vi "ERIO WIN Initialize all Process Variables.vi"(8 "error in (no error)":errorcluster, 9 "Tag Update Values":T1[](array[typedef]), 11 "EEISysLink.lvclass In":refnum<class "EEISysLink.lvclass">) -> (0 "error out":errorcluster, 3 "EEISysLink.lvclass Out":refnum<class "EEISysLink.lvclass">)   [LabVIEW 2017]
doc: "Will initialize all process variables on SystemLink in this ERIO evaluation cloud demo. This includes supervisory and worker types. This prepares the whole demo to run properly. \n\nNOTE: This Windows supervisor program must be run first before the sbRIO process target to properly initialize process variables and enable correct simulation operation. \n\nJames Tillett P.E.\nEndeavor Engineering Inc.\nwww.endeavoreng.com"
uses:
  Class EEISysLink/EEISysLink.lvclass
  Class EEISysLink/Controls/SL Tag Value.ctl
  Class EEISysLink/Controls/SL Tag Data Type.ctl
  Class EEISysLink/Controls/SL Tag Scope.ctl
  Class EEISysLink/Controls/SL Tag Type.ctl
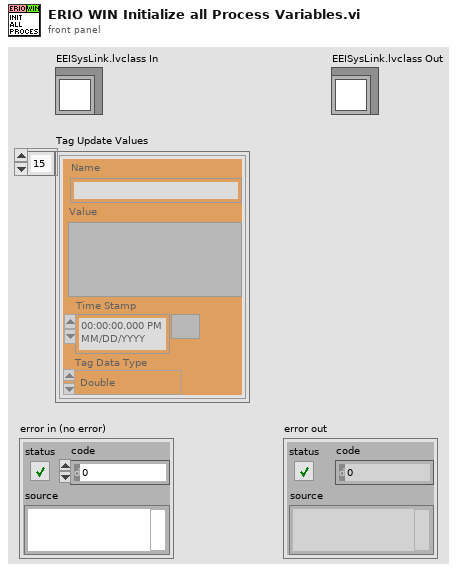
[diagram p1: front panel]
types:
  T1 = typedef "SL Tag Value.ctl" = cluster{"Value":variant, "Time Stamp":timestamp, "Tag Data Type":T2, "Name":string}
  T2 = typedef "EEISysLink.lvclass/SL Tag Data Type.ctl" = enum16{"Double", "Integer", "String", "Boolean", "Waveform"}
  T3 = typedef "EEISysLink.lvclass/SL Tag Type.ctl" = enum16{"All", "Supervisor", "Worker"}
  T4 = typedef "EEISysLink.lvclass/SL Tag Scope.ctl" = enum16{"Local", "Server"}
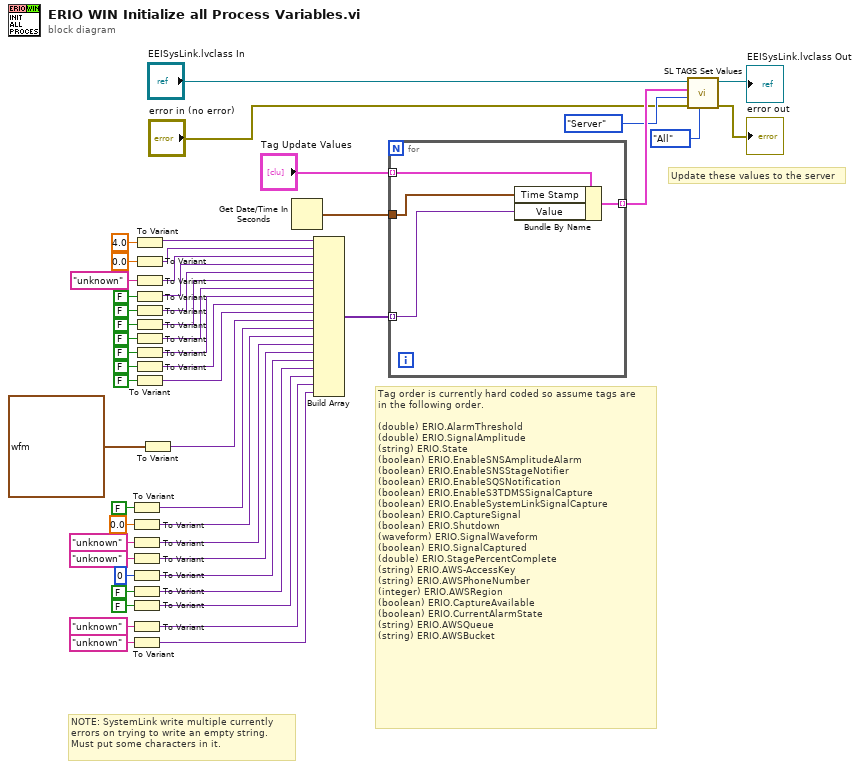
[diagram p0: block diagram]
diagram:
  # "NOTE: SystemLink write multiple currently\nerrors on trying to write an empty string.\nMust put some characters in it."
  # "Update these values to the server"
  # "Tag order is currently hard coded so assume tags are\nin the following order. \n\n(double) ERIO.AlarmThreshold\n(double) ERIO.SignalAmplitude\n(string) ERIO.State\n(boolean) ERIO.EnableSNSAmplitudeAlarm\n(boolean) ERIO.EnableSNSStageNotifier\n(boolean) ERIO.EnableSQSNotification\n(boolean) ERIO.EnableS3TDMSSignalCapture\n(boolean) ERIO.EnableSystemLinkSignalCapture\n(boolean) ERIO.CaptureSignal\n(boolean) ERIO.Shutdown\n(waveform) ERIO.SignalWaveform\n(boolean) ERIO.SignalCaptured\n(double) ERIO.StagePercentComplete\n(string) ERIO.AWS-AccessKey\n(string) ERIO.AWSPhoneNumber\n(integer) ERIO.AWSRegion\n(boolean) ERIO.CaptureAvailable\n(boolean) ERIO.CurrentAlarmState\n(string) ERIO.AWSQueue\n(string) ERIO.AWSBucket"
  n1 = To Variant(anything=FALSE) -> (Variant=w17:variant)
  n2 = To Variant(anything=0.0) -> (Variant=w15:variant)
  n3 = To Variant(anything="unknown") -> (Variant=w14:variant)
  n4 = To Variant(anything="unknown") -> (Variant=w13:variant)
  n5 = To Variant(anything=0) -> (Variant=w12:variant)
  n6 = To Variant(anything=FALSE) -> (Variant=w6:variant)
  n7 = To Variant(anything=FALSE) -> (Variant=w5:variant)
  n8 = To Variant(anything="unknown") -> (Variant=w2:variant)
  n9 = To Variant(anything="unknown") -> (Variant=w1:variant)
  n10 = To Variant(anything=4.0) -> (Variant=w30:variant)
  n11 = To Variant(anything=0.0) -> (Variant=w29:variant)
  n12 = To Variant(anything="unknown") -> (Variant=w28:variant)
  n13 = To Variant(anything=FALSE) -> (Variant=w27:variant)
  n14 = To Variant(anything=FALSE) -> (Variant=w26:variant)
  n15 = To Variant(anything=FALSE) -> (Variant=w25:variant)
  n16 = To Variant(anything=FALSE) -> (Variant=w24:variant)
  n17 = To Variant(anything=FALSE) -> (Variant=w23:variant)
  n18 = To Variant(anything=FALSE) -> (Variant=w22:variant)
  n19 = To Variant(anything=FALSE) -> (Variant=w21:variant)
  n20 = To Variant(anything=waveform(dbl) {"t0"=timestamp(0 s since 1904-01-01), "dt"=1.0, "Y"=[]} ("analog waveform")) -> (Variant=w19:variant)
  n21 = Get Date/Time In Seconds() -> (seconds since 1Jan1904=w49:timestamp)
  n22 = Build Array(w30, w29, w28, w27, w26, w25, w24, w23, w22, w21, w19, w17, w15, w14, w13, w12, w6, w5, w2, w1) -> (w48:variant[])
  n23 = for {
    tunnel: "Tag Update Values" -> [w54] mode=indexing
    tunnel: w49 -> [w53]
    tunnel: w48 -> [w52] mode=indexing
    tunnel: [w51] -> w47 mode=indexing
    n24 = Bundle By Name(cluster=w54, "Time Stamp"=w53, "Value"=w52) -> (w51:T1)
  }
  n25 = call-dynamic "SL TAGS Set Values.vi"("Tag Type"=SL_Tag_Type."All", "error in (no error)"="error in (no error)", "Tag Scope"=SL_Tag_Scope."Server", "Tag Update Values"=w47, "EEISysLink in"="EEISysLink.lvclass In") -> ("error out"=→"error out":errorcluster, "EEISysLink out"=→"EEISysLink.lvclass Out":refnum<class "EEISysLink.lvclass">)  [unwired: 5 in]
